vi "Write ApplicationRef.vi"(8 "error in (no error)":errorcluster, 10 "Application":refnum<vi>, 11 "Test Runner in":refnum<class "Test Runner.lvclass">) -> (0 "error out":errorcluster, 3 "Test Runner out":refnum<class "Test Runner.lvclass">)   [LabVIEW 2020, in "Caraya.lvlib" / "Test Runner.lvclass"]
uses:
  Test Runner.lvclass
  Test Runner.lvclass/Test Runner.ctl
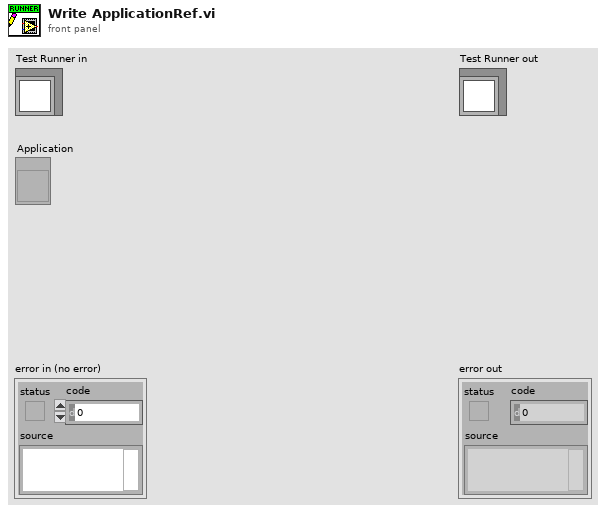
[diagram p1: front panel]
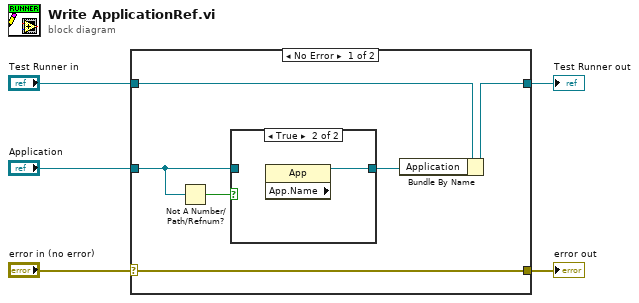
[diagram p0: block diagram]
diagram:
  n1 = case shown="No Error" "error in (no error)" {
    selector: "error in (no error)" -> [w11 w14]
    tunnel: [w11 w14] -> w4
    tunnel: [w7 w15] -> w2
    tunnel: "Test Runner in" -> [w8 w15]
    tunnel: "Application" -> [w9 _]
    frame No Error {
      n2 = Not A Number/Path/Refnum?(number/path/refnum=w9) -> (NaN/Path/Refnum?=w10:bool)
      n3 = case shown="True" w10 {
        tunnel: w9 -> [w12 _]
        tunnel: [w12 w13] -> w6
        frame False {
        }
        frame True {
          n4 = property class="App" props=["App.Name"]() -> (reference out=w13:refnum<vi>)  [unwired: 2 in, 2 out]
        }
      }
      n5 = Bundle By Name(cluster=w8, "Application"=w6) -> (w7:refnum<class "Test Runner.lvclass">)
    }
    frame Error {
    }
  }
  "error out" <- w4
  "Test Runner out" <- w2
